vi "VI_1.vi"() -> ()   [LabVIEW 2020]
panel:
  in  "Unit":bool
  out "Fahrenheit":dbl(slide) scale=0.0..100.0
  out "Celsius":dbl(slide) scale=0.0..100.0
  in  "Temperature":dbl
  in  "Operation":T1(ring)
  out "Answer":dbl
  in  "New":dbl
  in  "Temporary":dbl
  # "When switch(unit) is on it converts celsius to fahrenheit.\nWhen switch(unit) is off it converts Fahrenheit to celsius."
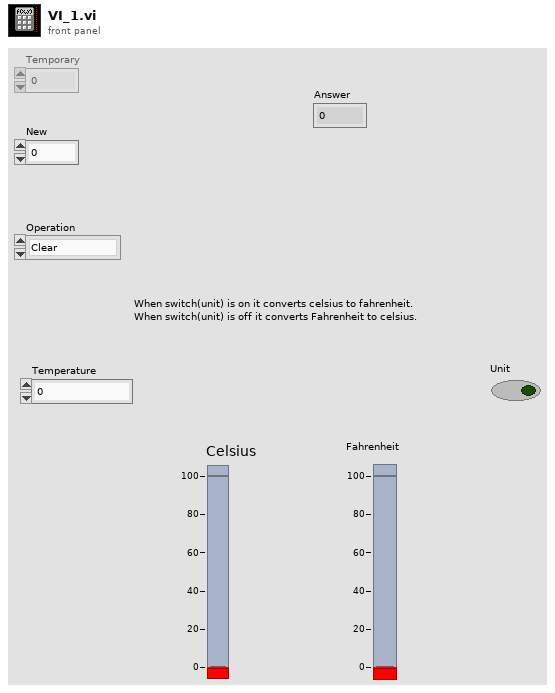
[diagram p1: front panel]
types:
  T1 = enum16{"Clear", "Addition", "Subtraction", "Multiplication", "Division", "Increment", "Decrement"}
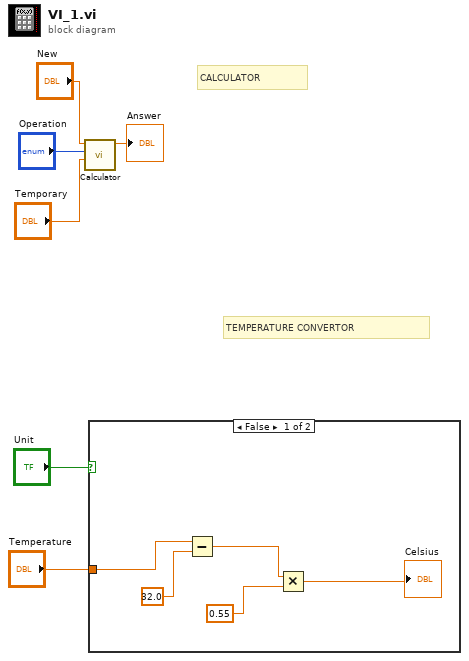
[diagram p0: block diagram]
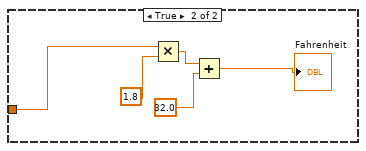
[diagram p2: hidden frame]
diagram:
  # "TEMPERATURE CONVERTOR"
  # "CALCULATOR"
  n1 = call "Calculator.vi"("Temporary"="Temporary", "Operation"="Operation", "New"="New") -> ("Numeric"=→"Answer":dbl)  [unwired: 8 in]
  n2 = case shown="False" "Unit" {
    tunnel: "Temperature" -> [w11 w13]
    frame False {
      n3 = Subtract(x=w11, y=32.0) -> (x-y=w9:dbl)
      n4 = Multiply(x=w9, y=0.55) -> (x*y=→"Celsius":dbl)
    }
    frame True {
      n5 = Multiply(x=w13, y=1.8) -> (x*y=w15:dbl)
      n6 = Add(x=w15, y=32.0) -> (x+y=→"Fahrenheit":dbl)
    }
  }
